vi "WPI_RelaySafetyUpdate.vi"(8 "error in (no error)":errorcluster, 11 "RelayDevRef":T1={"DevStatus"={"status"=FALSE, "code"=0, "source"=""}, "Relay Channel"=enum."Relay 2", "Relay Direction"=enum."Both directions"}) -> (0 "error out":errorcluster, 3 "RelayDevRef":T1={"DevStatus"={"status"=FALSE, "code"=0, "source"=""}, "Relay Channel"=enum."Relay 2", "Relay Direction"=enum."Both directions"})   [LabVIEW 2017]
doc: "Updates the safety output for Relays. When Safety Ouput has been enabled, this VI must be called in a loop that is faster than the <B>timeout</B> value of Safety Config VI. Otherwise the Relay output will be suspended until the next time Relay is updated.\n\nThis software is licensed. Open the labview\\readme\\WPI Robotics Library Open Source License.txt file for more information."
uses:
  <vilib>/Rock Robotics/WPI/Relay/WPI_RelayDevRef.ctl
  <vilib>/Rock Robotics/SystemInterfaces/DIO/FPGA_DIORelayChannel.ctl
  <vilib>/Rock Robotics/WPI/Relay/WPI_RelayDirection.ctl
  <vilib>/Rock Robotics/WPI/SafetyOutput/WPI_SafetyOutputCheckMenu.ctl
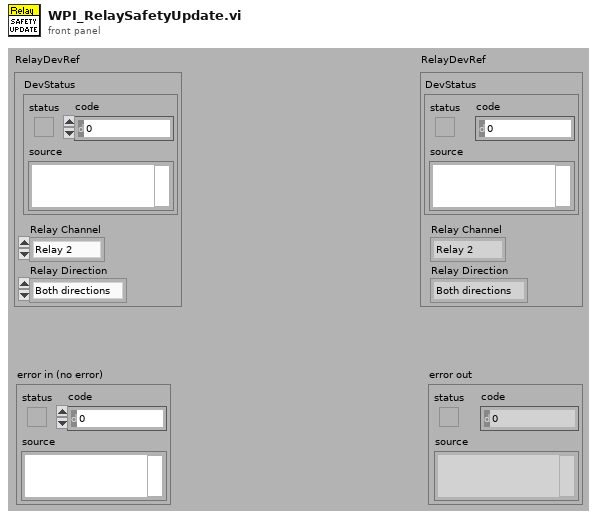
[diagram p1: front panel]
types:
  T1 = typedef "WPI_RelayDevRef.ctl" = cluster{"DevStatus":errorcluster, "Relay Channel":T2, "Relay Direction":T3}
  T2 = typedef "FPGA_DIORelayChannel.ctl" = enum8{"Relay 0", "Relay 1", "Relay 2", "Relay 3", "Invalid"}
  T3 = typedef "WPI_RelayDirection.ctl" = enum16{"Both directions", "Forward only", "Reverse only"}
  T4 = typedef "WPI_SafetyOutputCheckMenu.ctl" = enum16{"test", "add", "remove", "update"}
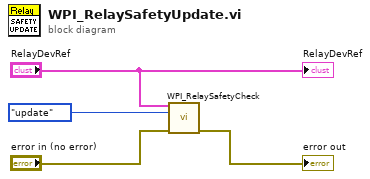
[diagram p0: block diagram]
diagram:
  n1 = call <vilib>:"WPI_RelaySafetyCheck.vi"("RelayDevRef"="RelayDevRef", "menu"=WPI_SafetyOutputCheckMenu."update", "error in (no error)"="error in (no error)") -> ("error out"=→"error out":errorcluster)  [unwired: 12 out]
  "RelayDevRef" <- "RelayDevRef"
